vi "MsgArrayToString.vi"(8 "error in":errorcluster, 10 "Message In":u8[](array[numeric]) format="%x") -> (0 "error out":errorcluster, 3 "Message Out":string)   [LabVIEW 2020, in "FirmataClient.lvlib"]
doc: "Transform a byte array into hex string where bytes are separated by dashes"
uses:
  FirmataClient.lvlib
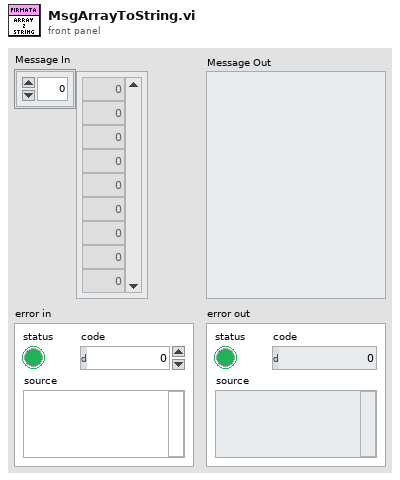
[diagram p1: front panel]
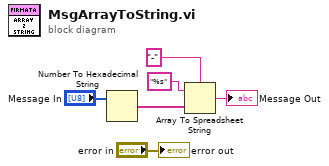
[diagram p0: block diagram]
diagram:
  n1 = Number To Hexadecimal String(2:"Message In") -> (0:w4:string[])  [unwired: 1 in]
  n2 = Array To Spreadsheet String(delimiter (Tab)="-", array=w4, 3:"%s" ("format string")) -> (spreadsheet string=→"Message Out":string)
  "error out" <- "error in"
